vi "myRIO_BRig_RT_dataCurrent_nCue1.vi"() -> (2 "output_nCue1":i32)   [LabVIEW 2014]
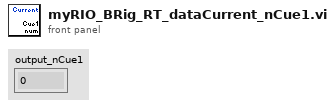
[diagram p1: front panel]
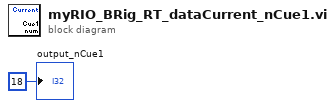
[diagram p0: block diagram]
diagram:
  "output_nCue1" <- 18 ("output_iBlock")
